vi "Configure.vi"(8 "error in (no error)":errorcluster, 10 "Channel  1":i32(ring) items=["A", "B"], 11 "VISA resource name":refnum<visa-resource-name>) -> (0 "error out":errorcluster, 3 "VISA resource name out":refnum<visa-resource-name>)   [LabVIEW 2019, in "CNT90.lvlib"]
uses:
  CNT90.lvlib
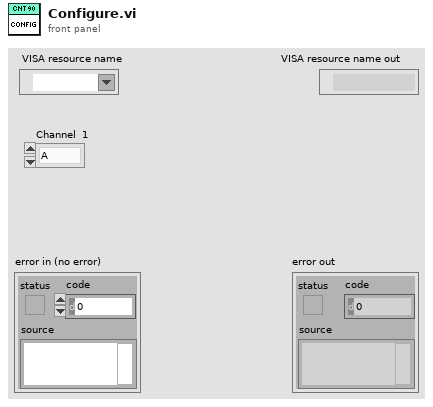
[diagram p1: front panel]
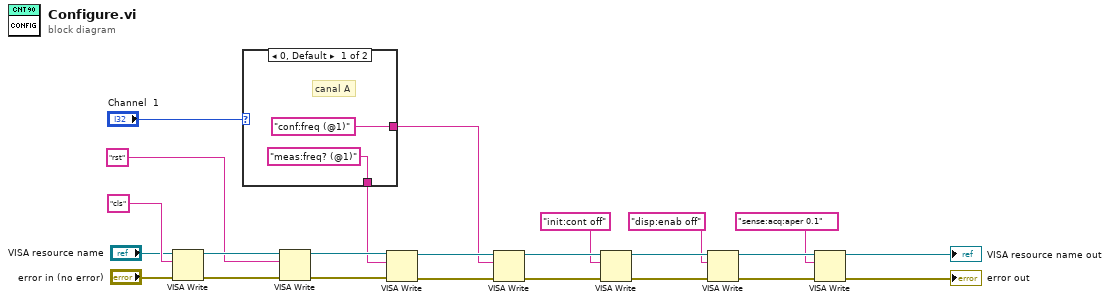
[diagram p0: block diagram]
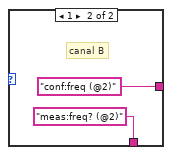
[diagram p2: hidden frame]
diagram:
  n1 = VISA Write(VISA resource name="VISA resource name", write buffer="cls", error in (no error)="error in (no error)") -> (VISA resource name out=w21:refnum<visa-resource-name>, error out=w24:errorcluster)  [unwired: 1 out]
  n2 = case shown="0, Default" "Channel  1" {
    tunnel: ["conf:freq (@1)" ("write buffer") "conf:freq (@2)" ("write buffer")] -> w9
    tunnel: ["meas:freq? (@1)" ("write buffer") "meas:freq? (@2)" ("write buffer")] -> w10
    frame 0, Default {
      # "canal A"
    }
    frame 1 {
      # "canal B"
    }
  }
  n3 = VISA Write(VISA resource name=w21, write buffer="rst", error in (no error)=w24) -> (VISA resource name out=w20:refnum<visa-resource-name>, error out=w23:errorcluster)  [unwired: 1 out]
  n4 = VISA Write(VISA resource name=w20, write buffer=w10, error in (no error)=w23) -> (VISA resource name out=w19:refnum<visa-resource-name>, error out=w22:errorcluster)  [unwired: 1 out]
  n5 = VISA Write(VISA resource name=w19, write buffer=w9, error in (no error)=w22) -> (VISA resource name out=w13:refnum<visa-resource-name>, error out=w14:errorcluster)  [unwired: 1 out]
  n6 = VISA Write(VISA resource name=w13, write buffer="init:cont off", error in (no error)=w14) -> (VISA resource name out=w12:refnum<visa-resource-name>, error out=w15:errorcluster)  [unwired: 1 out]
  n7 = VISA Write(VISA resource name=w12, write buffer="disp:enab off", error in (no error)=w15) -> (VISA resource name out=w11:refnum<visa-resource-name>, error out=w16:errorcluster)  [unwired: 1 out]
  n8 = VISA Write(VISA resource name=w11, write buffer="sense:acq:aper 0.1", error in (no error)=w16) -> (VISA resource name out=→"VISA resource name out":refnum<visa-resource-name>, error out=→"error out":errorcluster)  [unwired: 1 out]
